vi "Exponential Integral.vi"(2 "n":i32, 3 "x":dbl format="%.2f") -> (1 "En(x)":dbl format="%.2f")   [LabVIEW 2017, in "NI_Gmath.lvlib"]
doc: "Computes the exponential integral function."
uses:
  <vilib>/gmath/NI_Gmath.lvlib
  <resource>/lvanlys.dll
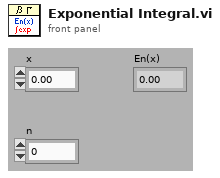
[diagram p1: front panel]
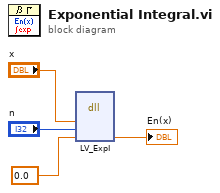
[diagram p0: block diagram]
diagram:
  n1 = dll-call lib="e:/builds/penguin/labview/branches/2017/dev/dist/resource/lvanlys.*" fn="LV_ExpI"("x"="x", "n"="n", "ExpI(x, n)"=0.0 ("expI")) -> ("ExpI(x, n)"=→"En(x)":dbl)  [unwired: 6 in, 2 out]
